vi "Auto_Routine_LeftTwoPieceTRAJ.vi"   [LabVIEW 2023]
uses:
  Arm2/ArmGetSetpointEnum.ctl
  Trajectory/TrajectoryGlobals.vi
  <vilib>/Rock Robotics/WPI/ThirdParty/JAS_Junk/TrajLib/Trajectory_Library.lvlib
types:
  T1 = typedef "ArmGetSetpointEnum.ctl" = enum16{"ArmFloorPickup", "ArmAmpDeposit", "ArmSpeakerShoot", "ArmStartPosition", "ArmRestPosition", "ArmSourceIntake", "ArmAwayShoot"}
  T2 = typedef "Trajectory_Library.lvlib/TRAJECTORY.ctl" = cluster{"TotalTImeSecs":dbl, "States":T3[]}
  T3 = typedef "Trajectory_Library.lvlib/TRAJ_STATE.ctl" = cluster{"TimeSeconds":dbl, "Velocity":dbl, "Acceleration":dbl, "POSE":T4, "Curvature":dbl}
  T4 = typedef "Trajectory_Library.lvlib/POSE2D.ctl" = cluster{"TRANSLATION":T5, "ROTATION":T6}
  T5 = typedef "Trajectory_Library.lvlib/TRANSLATION2D.ctl" = cluster{"X":dbl, "Y":dbl}
  T6 = typedef "Trajectory_Library.lvlib/ROTATION2D.ctl" = cluster{"VALUE":dbl, "COS":dbl, "SIN":dbl}
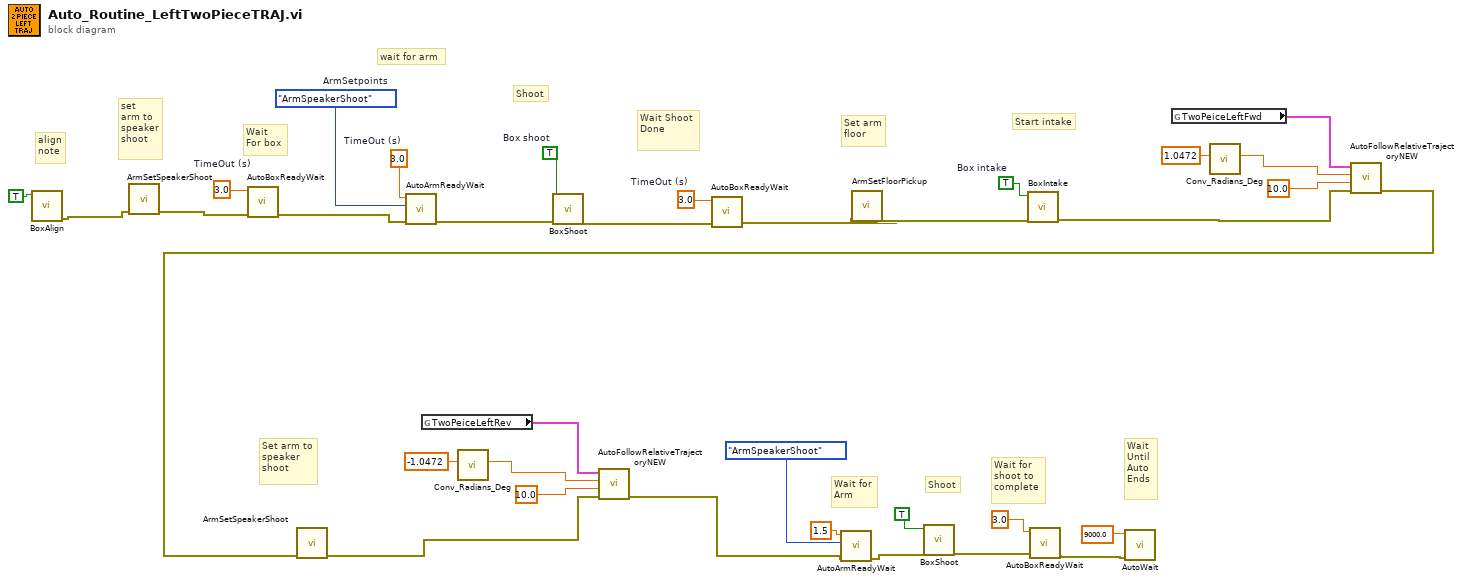
[diagram p0: block diagram]
diagram:
  w24 = 3.0  # TimeOut (s)
  w34 = TRUE  # Box intake
  w33 = TRUE  # Box shoot
  w32 = ArmGetSetpointEnum."ArmSpeakerShoot"  # ArmSetpoints
  w31 = 3.0  # TimeOut (s)
  w27 = 3.0  # TimeOut (s)
  # "Wait\nUntil\nAuto \nEnds"
  # "Wait for\nshoot to\ncomplete"
  # "Shoot"
  # "Wait for\nArm"
  # "Set arm to\nspeaker \nshoot"
  # "Start intake"
  # "Set arm\nfloor"
  # "Wait Shoot\nDone"
  # "Shoot"
  # "Wait\nFor box"
  # "set \narm to\nspeaker\nshoot"
  # "align\nnote"
  # "wait for arm"
  n1 = call "BoxAlign.vi"("box align"=TRUE) -> ("error out"=w25:errorcluster)  [unwired: 10 in]
  n2 = call "ArmSetSpeakerShoot.vi"("error in (no error)"=w25) -> ("error out"=w23:errorcluster)  [unwired: 10 in]
  n3 = call "AutoBoxReadyWait.vi"("error in (no error)"=w23, "TimeOut (s)"=w24) -> ("error out"=w22:errorcluster)  [unwired: 9 in]
  n4 = call "AutoArmReadyWait.vi"("error in (no error)"=w22, "ArmSetpoints"=w32, "TimeOut (s)"=w31) -> ("error out"=w28:errorcluster)  [unwired: 8 in]
  n5 = global read "TrajectoryGlobals.vi" "TwoPeiceLeftRev"() -> (w7:T2)
  n6 = call <vilib>:"Conv_Radians_Deg.vi"("Radians"=-1.0472) -> ("Degrees"=w5:dbl)  [unwired: 10 in]
  n7 = call "BoxShoot.vi"("error in (no error)"=w28, "Box shoot"=w33) -> ("error out"=w29:errorcluster)  [unwired: 9 in]
  n8 = call "AutoBoxReadyWait.vi"("error in (no error)"=w29, "TimeOut (s)"=w27) -> ("error out"=w21:errorcluster)  [unwired: 9 in]
  n9 = call "ArmSetFloorPickup.vi"("error in (no error)"=w21) -> ("error out"=w30:errorcluster)  [unwired: 10 in]
  n10 = call "BoxIntake.vi"("error in (no error)"=w30, "Box intake"=w34) -> ("error out"=w20:errorcluster)  [unwired: 9 in]
  n11 = global read "TrajectoryGlobals.vi" "TwoPeiceLeftFwd"() -> (w19:T2)
  n12 = call <vilib>:"Conv_Radians_Deg.vi"("Radians"=1.0472) -> ("Degrees"=w17:dbl)  [unwired: 10 in]
  n13 = call "AutoFollowRelativeTrajectoryNEW.vi"("error in (no error)"=w20, "TimeOut (s)"=10.0, "End Orientation"=w17, "Trajectory"=w19) -> ("error out"=w15:errorcluster)  [unwired: 7 in]
  n14 = call "ArmSetSpeakerShoot.vi"("error in (no error)"=w15) -> ("error out"=w3:errorcluster)  [unwired: 10 in]
  n15 = call "AutoFollowRelativeTrajectoryNEW.vi"("error in (no error)"=w3, "TimeOut (s)"=10.0, "End Orientation"=w5, "Trajectory"=w7) -> ("error out"=w2:errorcluster)  [unwired: 7 in]
  n16 = call "AutoArmReadyWait.vi"("error in (no error)"=w2, "ArmSetpoints"=ArmGetSetpointEnum."ArmSpeakerShoot", "TimeOut (s)"=1.5) -> ("error out"=w10:errorcluster)  [unwired: 8 in]
  n17 = call "BoxShoot.vi"("error in (no error)"=w10, "Box shoot"=TRUE) -> ("error out"=w13:errorcluster)  [unwired: 9 in]
  n18 = call "AutoBoxReadyWait.vi"("error in (no error)"=w13, "TimeOut (s)"=3.0) -> ("error out"=w1:errorcluster)  [unwired: 9 in]
  n19 = call "AutoWait.vi"("error in (no error)"=w1, "TimeOut (s)"=9000.0) -> ()  [unwired: 9 in, 1 out]
